vi "Set Flowrate.vi"() -> ()   [LabVIEW 2017]
panel:
  in  "Flowrate":u32
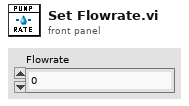
[diagram p1: front panel]
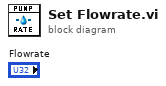
[diagram p0: block diagram]
diagram:
